vi "UpdateSelectedProperty.vi"(8 "error in (no error)":errorcluster, 11 "Highland T564 DDG in":refnum<class "Highland T564 DDG.lvclass">) -> (0 "error out":errorcluster, 3 "Highland T564 DDG out":refnum<class "Highland T564 DDG.lvclass">)   [LabVIEW 2020, in "Highland T564 DDG.lvclass"]
doc: "Update the 'SelectedProperty' value in the 'Settings' cluster"
uses:
  Highland T564 DDG.lvclass
  C:/GEECS/Developers Version/source/Device Drivers/shared/MetaDriver_v1/MetaDriver_v1.lvclass
  Highland T564 DDG.lvclass/Highland T564 DDG.ctl
  shared/MetaDriver_v1/MetaDriver_v1.lvclass
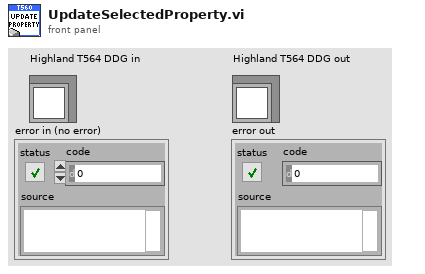
[diagram p1: front panel]
types:
  T1 = typedef "Highland T564 DDG.lvclass/settings Highland T560 DDG_TypDef.ctl" = cluster{"VisaResource":string, "BaudRate":u32, "Save":enum16{"off", "on"}, "LocalSavingPath":path, "Trigger":T2, "Channel1":T6, "Channel2":T6, "Channel3":T6, "Channel4":T6, "Simulation":T9}
  T2 = typedef "Trigger.ctl" = cluster{"Divisor":T3, "Level":T3, "Impedance":T4, "Source":T5}
  T3 = typedef "Choice01.ctl" = cluster{"Value":dbl, "Min":dbl, "Max":dbl, "StepSize":dbl, "Tolerance":dbl, "ValueActual":dbl}
  T4 = typedef "TriggerImpedance.ctl" = enum16{"10KOhm", "50Ohms"}
  T5 = typedef "TriggerSource.ctl" = enum16{"Rising", "Falling", "Internal 80MHz", "Internal DDS", "Remote", "Disabled"}
  T6 = typedef "Channel.ctl" = cluster{"Polarity":T7, "ChannelOn":enum16{"off", "on"}, "Delay":T3, "Width":T3, "ChannelName":T8}
  T7 = typedef "Choice83.ctl" = enum16{"Direct", "Inverted"}
  T8 = typedef "Choice84.ctl" = enum16{"Null", "A", "B", "C", "D", "Trigger"}
  T9 = typedef "OnOffTypeDef.ctl" = enum16{"off", "on"}
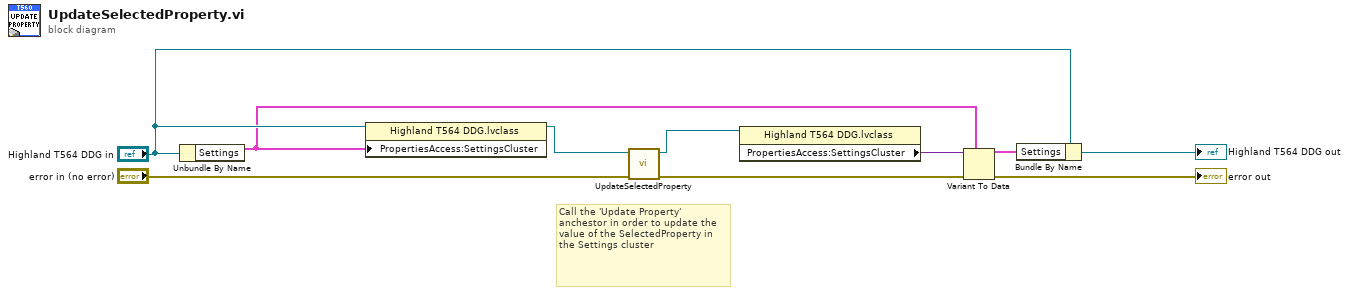
[diagram p0: block diagram]
diagram:
  # "Call the 'Update Property' anchestor in order to update the value of the SelectedProperty in the Settings cluster"
  n1 = Unbundle By Name("Highland T564 DDG in") -> ("Settings"=w7:T1)
  n2 = property class="Highland T564 DDG.lvclass"(reference="Highland T564 DDG in", "PropertiesAccess:SettingsCluster"=w7) -> (reference out=w3:refnum<class "Highland T564 DDG.lvclass">)  [unwired: 1 in, 1 out]
  n3 = call-parent "UpdateSelectedProperty.vi"("error in (no error)"="error in (no error)", "MetaDriver_v1 in"=w3) -> ("error out"=w1:errorcluster, "MetaDriver_v1 out"=w2:refnum<class "Highland T564 DDG.lvclass">)  [unwired: 8 in]
  n4 = property class="Highland T564 DDG.lvclass"(reference=w2) -> ("PropertiesAccess:SettingsCluster"=w5:variant)  [unwired: 1 in, 2 out]
  n5 = Variant To Data(error in=w1, type=w7, Variant=w5) -> (data=w8:T1, error out=→"error out":errorcluster)
  n6 = Bundle By Name(cluster="Highland T564 DDG in", "Settings"=w8) -> (→"Highland T564 DDG out":refnum<class "Highland T564 DDG.lvclass">)
